vi "RGTWordImageInTable.vi"() -> ()   [LabVIEW 2010]
uses:
  <vilib>/Utility/NIReport.llb/Append Text Table to Report (wrap).vi
  <vilib>/addons/_office/word.llb/Word Edit Cell (path).vi
  <vilib>/Utility/NIReport.llb/NI_report.lvclass
  <vilib>/Utility/NIReport.llb/Word/NI_Word.lvclass
  <vilib>/addons/_office/NI_ReportGenerationToolkit.lvlib
panel:
  in  "Path":path
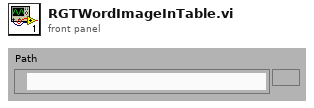
[diagram p1: front panel]
types:
  T1 = enum16{"maximized", "minimized", "normal", "no change"}
  T2 = enum16{"Standard Report", "HTML", "Word", "Excel"}
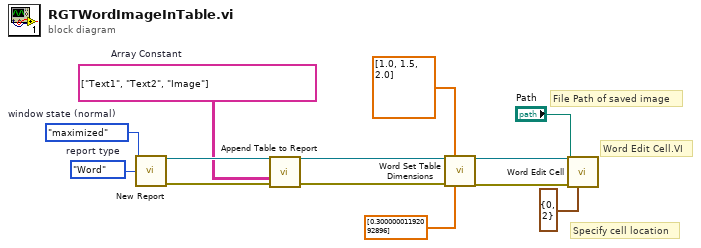
[diagram p0: block diagram]
diagram:
  w5 = T1."maximized"  # window state (normal)
  w7 = T2."Word"  # report type
  w11 = string[][] [["Text1", "Text2", "Image"]]  # Array Constant
  # "Specify cell location"
  # "File Path of saved image"
  # "Word Edit Cell.VI"
  n1 = call <vilib>:"New Report.vi"("window state (normal)"=w5, "report type"=w7) -> ("report out"=w13:refnum<class "NI_report.lvclass">, "error out"=w12:errorcluster)  [unwired: 4 in, 8 out]
  n2 = call-poly <vilib>:"Append Table to Report.vi"("report in"=w13, "text data"=w11, "error in (no error)"=w12) -> ("report out"=w9:refnum<class "NI_report.lvclass">, "error out"=w10:errorcluster)  [unwired: 6 in, 5 out]
  n3 = call <vilib>:"Word Set Table Dimensions.vi"("report in"=w9, "table column widths"=sgl[] [1.0, 1.5, 2.0], "error in (no error)"=w10, "table row heights"=sgl[] [0.3]) -> ("report out"=w4:refnum<class "NI_report.lvclass">, "error out"=w3:errorcluster)  [unwired: 2 in, 8 out]
  n4 = call-poly <vilib>:"Word Edit Cell.vi"("report in"=w4, "value"="Path", "error in (no error)"=w3, "start (0, 0)"=cluster{"row":i32, "column":i32} {"row"=0, "column"=2}) -> ()  [unwired: 10 in, 2 out]
